vi "CRYDisplay Unicode String Text.vi"(5 "Interpret as Unicode (T)":bool, 6 "error in":errorcluster, 8 "String Value":string, 9 "String Control Reference":refnum<vi>) -> (0 "error out":errorcluster, 3 "String Control Reference":refnum<vi>)   [LabVIEW 2013]
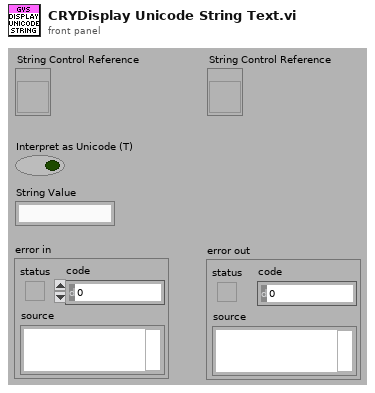
[diagram p1: front panel]
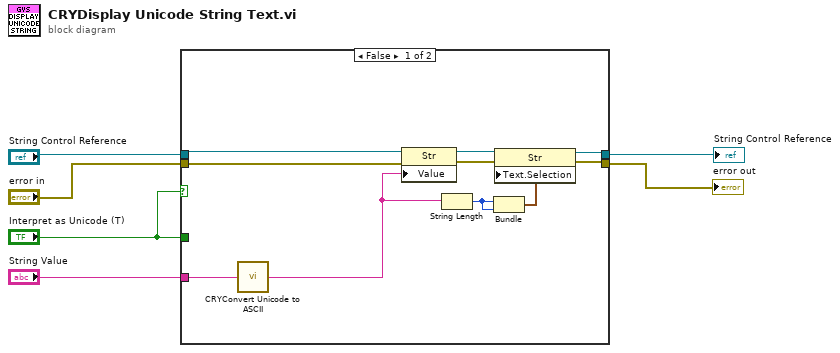
[diagram p0: block diagram]
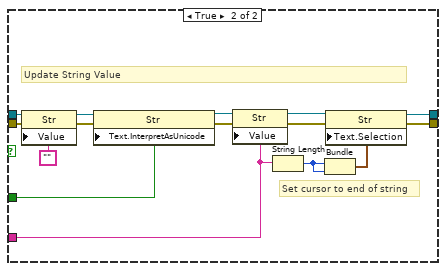
[diagram p2: hidden frame]
diagram:
  n1 = case shown="False" "Interpret as Unicode (T)" {
    tunnel: "String Control Reference" -> [w12 w31]
    tunnel: "error in" -> [w9 w30]
    tunnel: "Interpret as Unicode (T)" -> [_ w29]
    tunnel: "String Value" -> [w8 w23]
    tunnel: [w10 w22] -> w3
    tunnel: [w11 w17] -> w2
    frame False {
      n2 = call "CRYConvert Unicode to ASCII.vi"("Unicode"=w8) -> ("ASCII"=w7:string)  [unwired: 4 in]
      n3 = property class="Str"(reference=w12, error in=w9, "Value"=w7) -> (reference out=w13:refnum<vi>, error out=w14:errorcluster)
      n4 = String Length(string=w7) -> (length=w15:i32)
      n5 = Bundle(w15, w15) -> (w16:cluster{i32, i32})  [unwired: 1 in]
      n6 = property class="Str"(reference=w13, error in=w14, "Text.Selection"=w16) -> (reference out=w11:refnum<vi>, error out=w10:errorcluster)
    }
    frame True {
      # "Update String Value"
      # "Set cursor to end of string"
      n7 = property class="Str"(reference=w31, error in=w30, "Value"="") -> (reference out=w19:refnum<vi>, error out=w26:errorcluster)
      n8 = property class="Str"(reference=w19, error in=w26, "Text.InterpretAsUnicode"=w29) -> (reference out=w28:refnum<vi>, error out=w27:errorcluster)
      n9 = property class="Str"(reference=w28, error in=w27, "Value"=w23) -> (reference out=w20:refnum<vi>, error out=w21:errorcluster)
      n10 = String Length(string=w23) -> (length=w24:i32)
      n11 = Bundle(w24, w24) -> (w25:cluster{i32, i32})  [unwired: 1 in]
      n12 = property class="Str"(reference=w20, error in=w21, "Text.Selection"=w25) -> (reference out=w17:refnum<vi>, error out=w22:errorcluster)
    }
  }
  "error out" <- w3
  "String Control Reference" <- w2
